vi "tlc_Play.vi"(8 "error in (no error)":errorcluster) -> (0 "error out":errorcluster, 3 "Stop?":bool)   [LabVIEW 2018]
doc: "This VI will perform the functionality for playing a Cue for the Theatre Light Controller."
uses:
  Controls/Play.ctl
  Modules/Cue/tlc_Cue_Information Command.ctl
  Controls/Cue State.ctl
  Modules/Timing/tlc_Timing Command Control.ctl
  Controls/tlc_User Interface Data Type.ctl
panel:
  # "Input Data"
  # "Internal Data"
  # "Output Data"
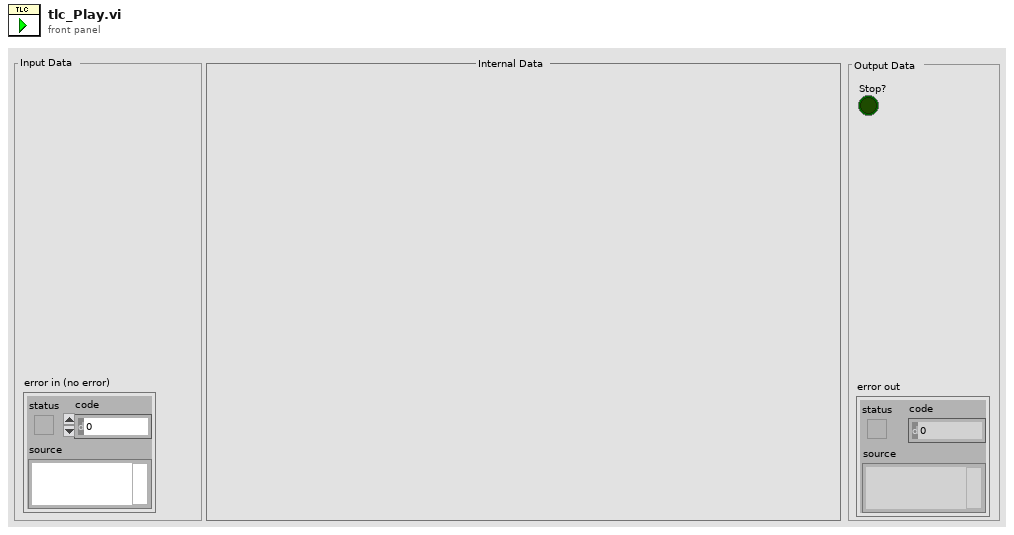
[diagram p1: front panel]
types:
  T1 = typedef "Play.ctl" = enum16{"Initialize", "Begin Play", "Load Cue", "Wait Time", "Fade Time", "Follow Time", "Check for Next Cue", "End Play"}
  T2 = typedef "tlc_Timing Command Control.ctl" = enum16{"Initialize", "Get Information", "Create", "Wait", "Fade", "Follow", "Shutdown"}
  T3 = typedef "Cue State.ctl" = cluster{"Increment":dbl, "Desired Color":u32}
  T4 = typedef "tlc_Cue_Information Command.ctl" = enum16{"Add Cue", "Delete Cue", "Get Cue Values", "Set Cue Values", "Swap", "Get Number of Cues", "Initialize", "Get Empty Cue"}
  T5 = typedef "tlc_User Interface Data Type.ctl" = enum16{"Initialize", "Initialize Front Panel", "Update Front Panel Channels", "Select Cue in Cue List", "Enable/Disable Front Panel Controls", "Update Cue List", "Stop"}
  T6 = typedef "tlc_Cue_Information.ctl" = cluster{"Cue Name":string, "Wait Time (s)":u32, "Fade Time (s)":u32, "Follow Time (s)":u32, "Channels":T7[][]}
  T7 = typedef "channel.ctl" = cluster{"Intensity":dbl, " Color":u32, "Channel":i32}
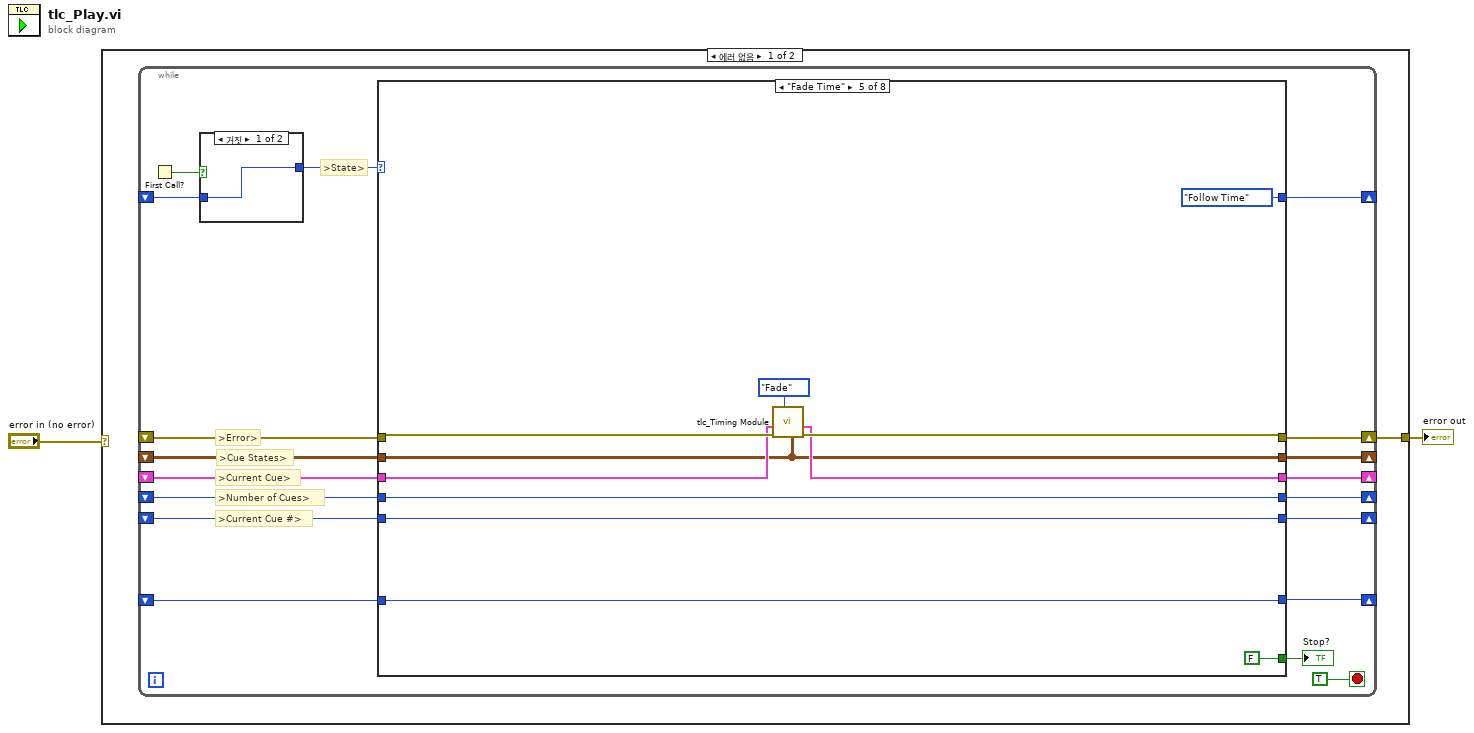
[diagram p0: block diagram]
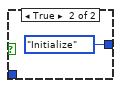
[diagram p2: hidden frame]
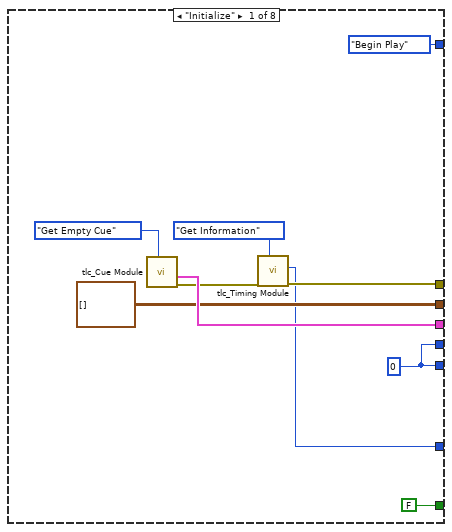
[diagram p3: hidden frame]
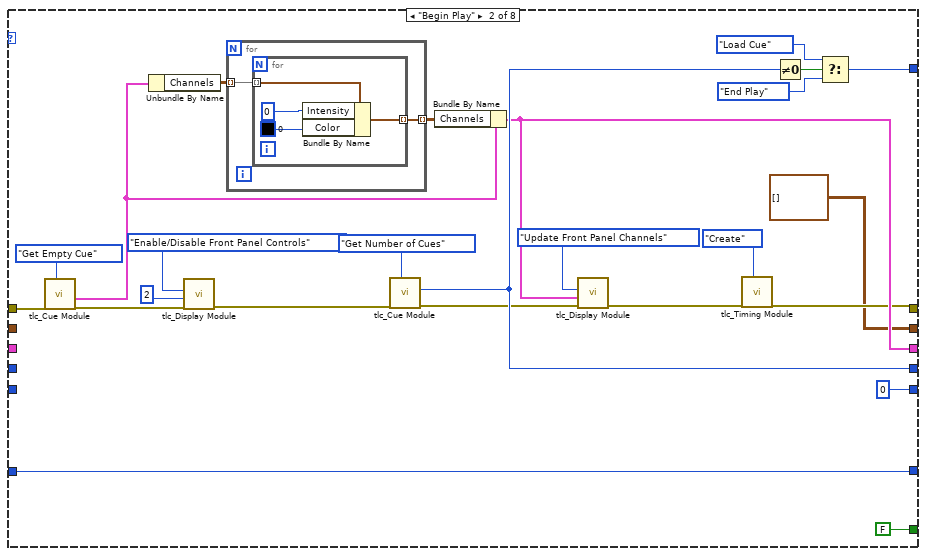
[diagram p4: hidden frame]
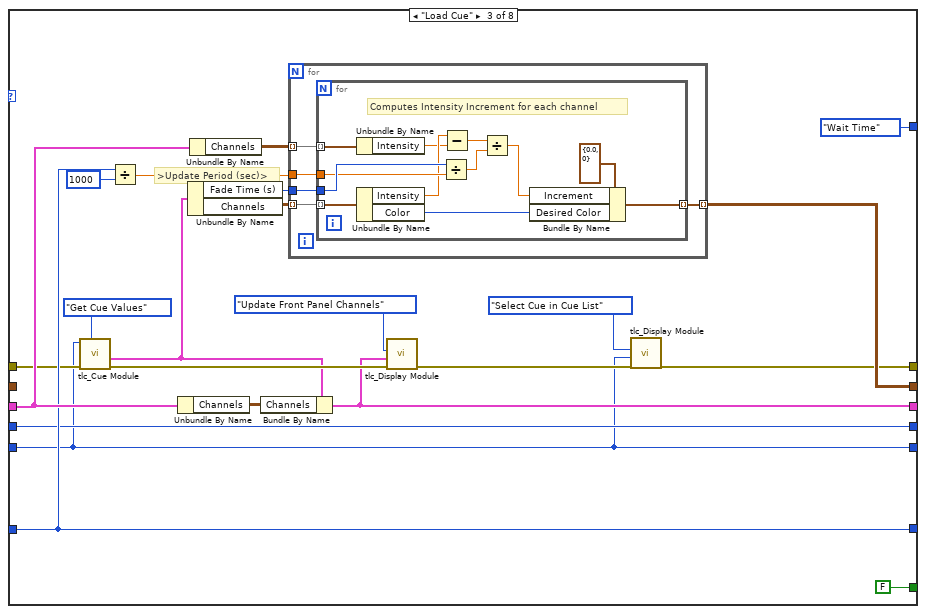
[diagram p5: hidden frame]
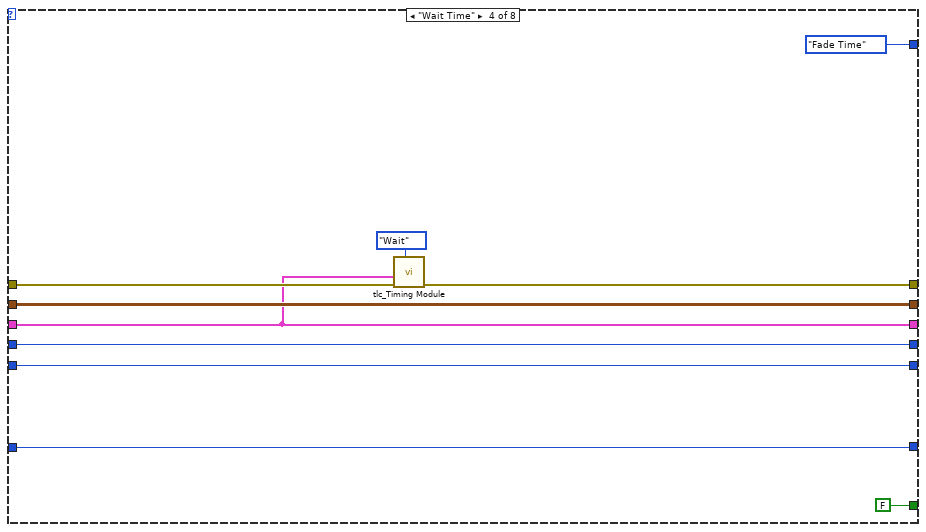
[diagram p6: hidden frame]
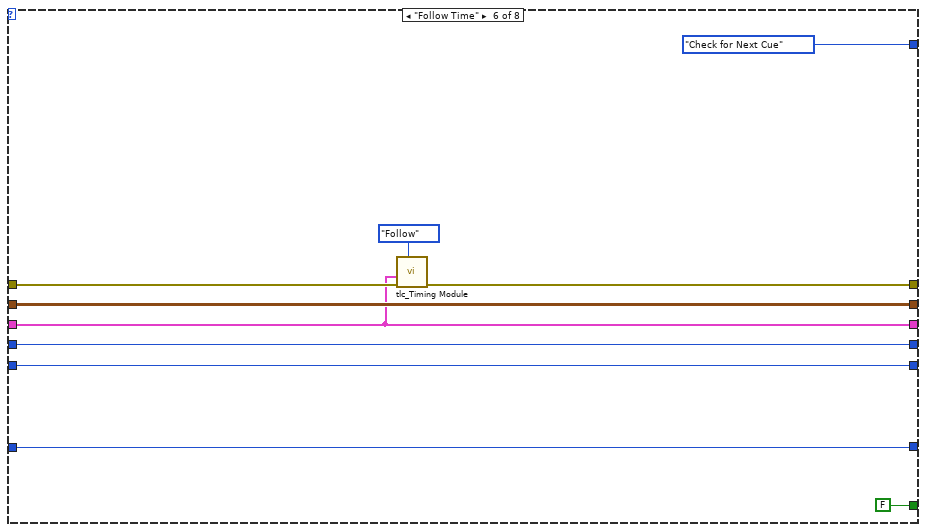
[diagram p7: hidden frame]
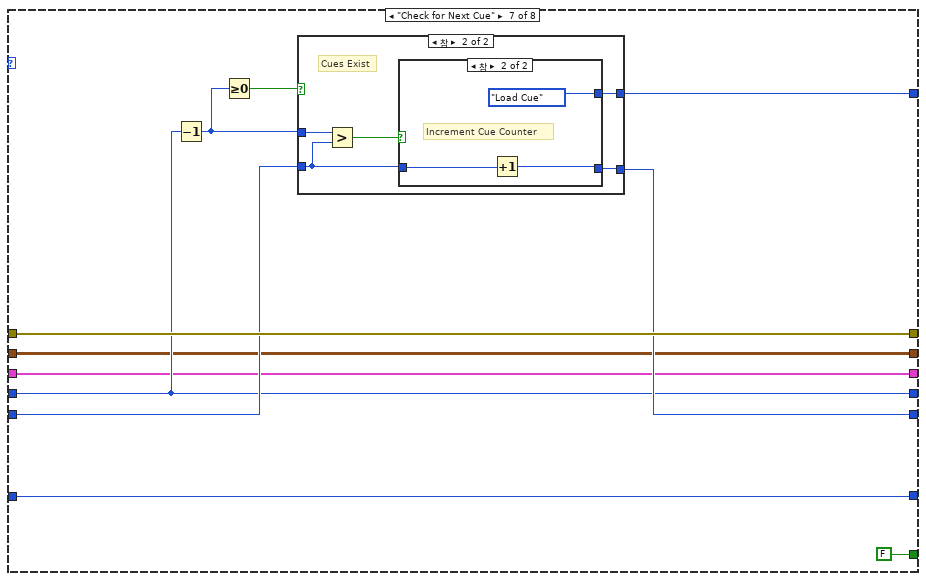
[diagram p8: hidden frame]
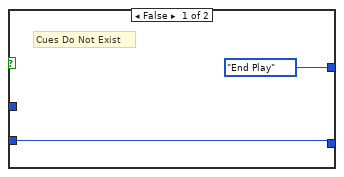
[diagram p9: hidden frame]
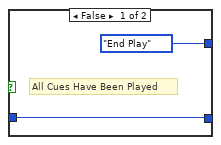
[diagram p10: hidden frame]
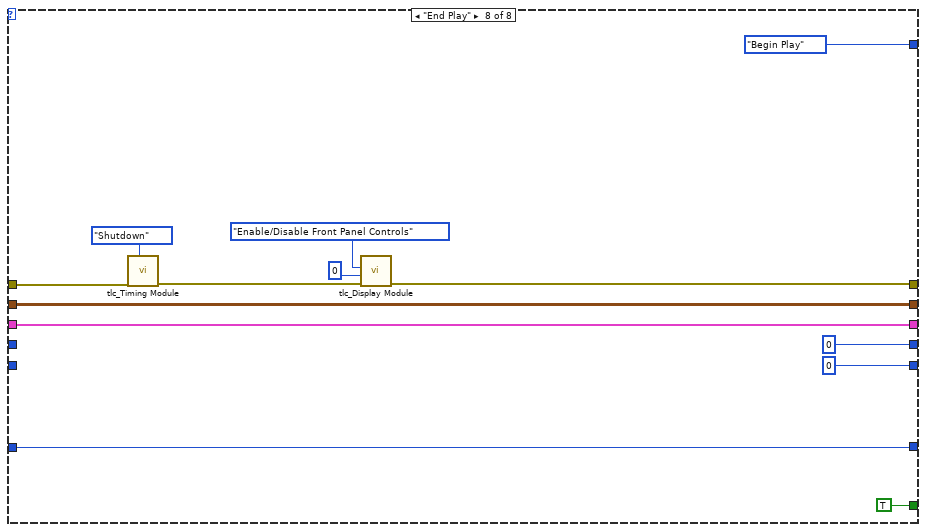
[diagram p11: hidden frame]
diagram:
  n1 = case shown="에러 없음" "error in (no error)" {
    selector: "error in (no error)" -> [_ w171]
    tunnel: [w3 w171] -> w2
    frame No Error {
      n2 = while {
        shift-right: [w20] -> _
        shift-left: _ -> [w9]
        shift-right: [w13] -> w3
        shift-left: _ -> [w21]
        shift-right: [w19] -> _
        shift-left: _ -> [w18]
        shift-right: [w14] -> _
        shift-left: _ -> [w17]
        shift-right: [w15] -> _
        shift-left: _ -> [w16]
        shift-right: [w8] -> _
        shift-left: _ -> [w7]
        shift-right: [w6] -> _
        shift-left: _ -> [w5]
        stop <- TRUE stop-if-true
        # ">Cue States>"
        # ">Error>"
        # ">Current Cue #>"
        # ">Number of Cues>"
        # ">State>"
        # ">Current Cue>"
        n3 = First Call?() -> (First Call?: T/F=w4:bool)
        n4 = case shown="거짓" w4 {
          tunnel: [w22 Play."Initialize"] -> w10
          tunnel: w9 -> [w22 _]
          frame False {
          }
          frame True {
          }
        }
        n5 = case shown="\"Fade Time\"" w10 {
          tunnel: [FALSE FALSE FALSE FALSE FALSE FALSE FALSE TRUE] -> w11
          tunnel: w21 -> [_ w43 w75 w107 w119 w128 w145 w163]
          tunnel: [w26 w36 w68 w106 w118 w127 w145 w161] -> w13
          tunnel: [Play."Begin Play" ("t") w55 Play."Wait Time" Play."Fade Time" ("t") Play."Follow Time" ("t") Play."Check for Next Cue" ("t") w142 Play."Begin Play"] -> w20
          tunnel: [w33 w44 w66 w113 w124 w134 w138 0 ("Number of Cues")] -> w19
          tunnel: w18 -> [_ _ w66 w113 w124 w134 w138 _]
          tunnel: [w30 w38 w70 w105 w117 w126 w137 w168] -> w14
          tunnel: w17 -> [_ _ w80 w105 w116 w126 w137 w168]
          tunnel: w16 -> [_ _ w65 w112 w123 w133 w140 _]
          tunnel: [w33 0 w65 w112 w123 w133 w143 0] -> w15
          tunnel: [w25 w50 w76 w108 w120 w129 w135 w164] -> w6
          tunnel: [T3[][] [] T3[][] [] w81 w109 w114 w130 w136 w165] -> w8
          tunnel: w7 -> [_ _ _ w109 w114 w130 w136 w165]
          tunnel: w5 -> [_ w50 w76 w108 w120 w129 w135 w164]
          frame "Initialize" {
            w33 = 0
            n6 = call "tlc_Cue Module.vi"("Command"=tlc_Cue_Information_Command."Get Empty Cue" ("Enum")) -> ("error out"=w27:errorcluster, "Cue Output"=w30:T6)  [unwired: 7 in, 1 out]
            n7 = call "tlc_Timing Module.vi"("Command"=tlc_Timing_Command_Control."Get Information", "error in (no error)"=w27) -> ("error out"=w26:errorcluster, "Update Rate Out"=w25:u32)  [unwired: 7 in, 1 out]
          }
          frame "Begin Play" {
            n8 = call "tlc_Cue Module.vi"("Command"=tlc_Cue_Information_Command."Get Empty Cue" ("Enum"), "error in (no error)"=w43) -> ("error out"=w42:errorcluster, "Cue Output"=w49:T6)  [unwired: 6 in, 1 out]
            n9 = Unbundle By Name(w49) -> ("Channels"=w53:T7[][])
            n10 = call "tlc_Display Module.vi"("error in (no error)"=w42, "Data"=2, "Data Type"=tlc_User_Interface_Data_Type."Enable/Disable Front Panel Controls") -> ("error out"=w41:errorcluster)  [unwired: 8 in]
            n11 = for {
              tunnel: w53 -> [w60] mode=indexing
              tunnel: [w59] -> w52 mode=indexing
              n12 = for {
                tunnel: w60 -> [w64] mode=indexing
                tunnel: [w61] -> w59 mode=indexing
                n13 = Bundle By Name(cluster=w64, "Intensity"=u32 0 ("Current Intensity"), "Color"=u32 0 ("Current Color")) -> (w61:T7)
              }
            }
            n14 = call "tlc_Cue Module.vi"("Command"=tlc_Cue_Information_Command."Get Number of Cues" ("Enum"), "error in (no error)"=w41) -> ("error out"=w40:errorcluster, "Number of Cues"=w44:i32)  [unwired: 6 in, 1 out]
            n15 = Bundle By Name(cluster=w49, "Channels"=w52) -> (w38:T6)
            n16 = call "tlc_Display Module.vi"("error in (no error)"=w40, "Data"=w38, "Data Type"=tlc_User_Interface_Data_Type."Update Front Panel Channels") -> ("error out"=w37:errorcluster)  [unwired: 8 in]
            n17 = call "tlc_Timing Module.vi"("Command"=tlc_Timing_Command_Control."Create", "error in (no error)"=w37) -> ("error out"=w36:errorcluster)  [unwired: 7 in, 2 out]
            n18 = Not Equal To 0?(x=w44) -> (x != 0?=w58:bool)
            n19 = Select(t=Play."Load Cue", s=w58, f=Play."End Play" ("t")) -> (s? t:f=w55:T1)
          }
          frame "Load Cue" {
            # ">Update Period (sec)>"
            n20 = call "tlc_Cue Module.vi"("Command"=tlc_Cue_Information_Command."Get Cue Values" ("Enum"), "error in (no error)"=w75, "Cue Index"=w65) -> ("error out"=w74:errorcluster, "Cue Output"=w72:T6)  [unwired: 5 in, 1 out]
            n21 = Divide(x=w76, y=u32 1000) -> (x/y=w77:dbl)
            n22 = Unbundle By Name(w80) -> ("Channels"=w79:T7[][])
            n23 = Unbundle By Name(w72) -> ("Fade Time (s)"=w83:u32, "Channels"=w84:T7[][])
            n24 = Unbundle By Name(w80) -> ("Channels"=w85:T7[][])
            n25 = Bundle By Name(cluster=w72, "Channels"=w79) -> (w70:T6)
            n26 = for {
              tunnel: w85 -> [w91] mode=indexing
              tunnel: w84 -> [w90] mode=indexing
              tunnel: w77 -> [w89]
              tunnel: w83 -> [w88]
              tunnel: [w87] -> w81 mode=indexing
              n27 = for {
                tunnel: w91 -> [w96] mode=indexing
                tunnel: w88 -> [w102]
                tunnel: w90 -> [w103] mode=indexing
                tunnel: w89 -> [w99]
                tunnel: [w93] -> w87 mode=indexing
                # "Computes Intensity Increment for each channel"
                n28 = Unbundle By Name(w96) -> ("Intensity"=w97:dbl)
                n29 = Unbundle By Name(w103) -> ("Intensity"=w98:dbl, "Color"=w94:u32)
                n30 = Divide(x=w102, y=w99) -> (x/y=w100:dbl)
                n31 = Subtract(x=w98, y=w97) -> (x-y=w101:dbl)
                n32 = Divide(x=w101, y=w100) -> (x/y=w95:dbl)
                n33 = Bundle By Name(cluster=T3 {"Increment"=0.0, "Desired Color"=0} ("Cue State"), "Increment"=w95, "Desired Color"=w94) -> (w93:T3)
              }
            }
            n34 = call "tlc_Display Module.vi"("error in (no error)"=w74, "Data"=w70, "Data Type"=tlc_User_Interface_Data_Type."Update Front Panel Channels") -> ("error out"=w69:errorcluster)  [unwired: 8 in]
            n35 = call "tlc_Display Module.vi"("error in (no error)"=w69, "Data"=w65, "Data Type"=tlc_User_Interface_Data_Type."Select Cue in Cue List") -> ("error out"=w68:errorcluster)  [unwired: 8 in]
          }
          frame "Wait Time" {
            n36 = call "tlc_Timing Module.vi"("Command"=tlc_Timing_Command_Control."Wait", "error in (no error)"=w107, "Cue Input"=w105) -> ("error out"=w106:errorcluster)  [unwired: 6 in, 2 out]
          }
          frame "Fade Time" {
            n37 = call "tlc_Timing Module.vi"("Cue States"=w114, "Command"=tlc_Timing_Command_Control."Fade", "error in (no error)"=w119, "Cue Input"=w116) -> ("error out"=w118:errorcluster, "Cue Output"=w117:T6)  [unwired: 5 in, 1 out]
          }
          frame "Follow Time" {
            n38 = call "tlc_Timing Module.vi"("Command"=tlc_Timing_Command_Control."Follow", "error in (no error)"=w128, "Cue Input"=w126) -> ("error out"=w127:errorcluster)  [unwired: 6 in, 2 out]
          }
          frame "Check for Next Cue" {
            n39 = Decrement(x=w138) -> (x-1=w139:i32)
            n40 = Greater Or Equal To 0?(x=w139) -> (x >= 0?=w141:bool)
            n41 = case shown="참" w141 {
              tunnel: [w147 w152] -> w143
              tunnel: [Play."End Play" ("t") w151] -> w142
              tunnel: w140 -> [w147 w148]
              tunnel: w139 -> [_ w149]
              frame False {
                # "Cues Do Not Exist"
              }
              frame True {
                # "Cues Exist"
                n42 = Greater?(x=w149, y=w148) -> (0:w150:bool)
                n43 = case shown="참" w150 {
                  tunnel: w148 -> [w153 w157]
                  tunnel: [w153 w156] -> w152
                  tunnel: [Play."End Play" ("t") Play."Load Cue" ("t")] -> w151
                  frame False {
                    # "All Cues Have Been Played"
                  }
                  frame True {
                    # "Increment Cue Counter"
                    n44 = Increment(x=w157) -> (x+1=w156:i32)
                  }
                }
              }
            }
          }
          frame "End Play" {
            n45 = call "tlc_Timing Module.vi"("Command"=tlc_Timing_Command_Control."Shutdown", "error in (no error)"=w163) -> ("error out"=w162:errorcluster)  [unwired: 7 in, 2 out]
            n46 = call "tlc_Display Module.vi"("error in (no error)"=w162, "Data"=0, "Data Type"=tlc_User_Interface_Data_Type."Enable/Disable Front Panel Controls") -> ("error out"=w161:errorcluster)  [unwired: 8 in]
          }
        }
        "Stop?" <- w11
      }
    }
    frame Error {
    }
  }
  "error out" <- w2
